vi "classification to module permissions.vi"(11 "channel classification":T1) -> (3 "view direction":enum32{"Read from HW", "Write to HW"}(radio))   [LabVIEW 2015, in "TDMS datalogger configuration.lvclass"]
uses:
  TDMS datalogger configuration.lvclass
  <vilib>/NI/Tag Bus Module Framework/channel/channel classification.ctl
  <vilib>/NI/Tag Bus Module Framework/channel/TBM channel.lvclass
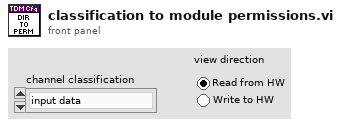
[diagram p1: front panel]
types:
  T1 = typedef "TBM channel.lvclass/channel classification.ctl" = enum16{"input data", "output data", "processing parameter", "processing result"}
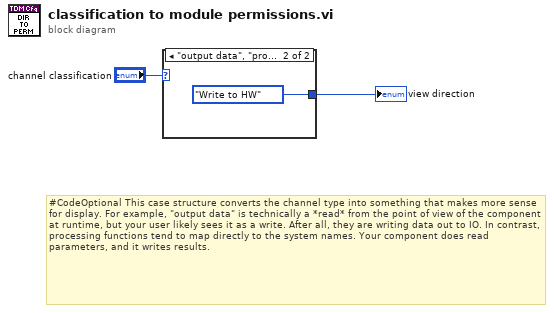
[diagram p0: block diagram]
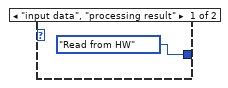
[diagram p2: hidden frame]
diagram:
  # "#CodeOptional This case structure converts the channel type into something that makes more sense for display. For example, \"output data\" is technically a *read* from the point of view of the component at runtime, but your user likely sees it as a write. After all, they are writing data out to IO. In contrast, processing functions tend to map directly to the system names. Your component does read parameters, and it writes results."
  n1 = case shown="\"output data\", \"processing parameter\"" "channel classification" {
    tunnel: [enum32{"Read from HW", "Write to HW"}."Read from HW" ("view direction") enum32{"Read from HW", "Write to HW"}."Write to HW" ("view direction")] -> w1
    frame "input data", "processing result" {
    }
    frame "output data", "processing parameter" {
    }
  }
  "view direction" <- w1
